vi "DSF.Engine.Plugin.Start.vi"(8 "error in (no error)":errorcluster, 11 "Plugin in":refnum<class "DSF.Engine.Plugin.lvclass">) -> (0 "error out":errorcluster, 3 "Plugin out":refnum<class "DSF.Engine.Plugin.lvclass">)   [LabVIEW 2017, in "DSF.Engine.lvlib" / "DSF.Engine.Plugin.lvclass"]
uses:
  DSF.Engine.Plugin.lvclass
  DSF.Engine.Plugin.lvclass/DSF.Engine.Plugin.ctl
  Timing/DSF.Engine.Timing.lvclass/DSF.Engine.Timing.ctl
  Transceiver/DSF.Engine.Transceiver Thread.lvclass
  Thread Pool/DSF.Engine.Pool.ID.lvclass
  Thread Parameters/Thread Parameters.lvclass
  Timing/DSF.Engine.Timing.lvclass
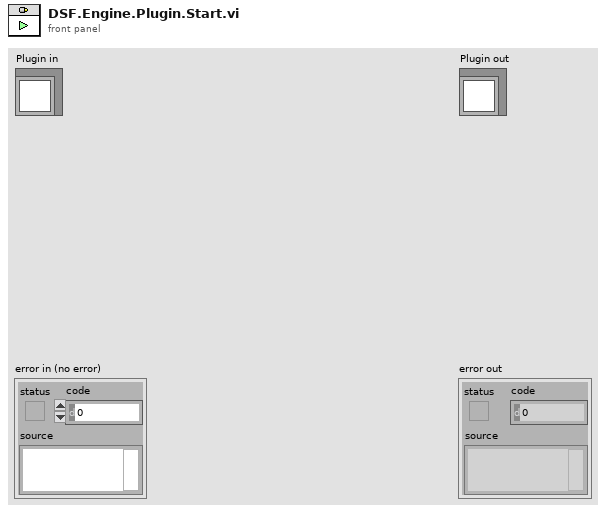
[diagram p1: front panel]
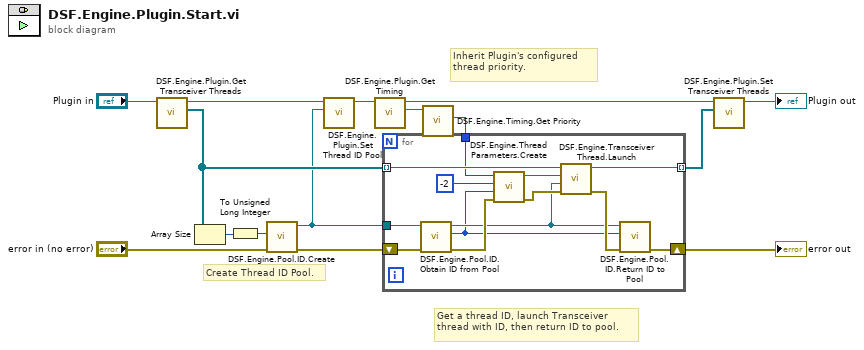
[diagram p0: block diagram]
diagram:
  # "Inherit Plugin's configured thread priority."
  # "Get a thread ID, launch Transceiver thread with ID, then return ID to pool."
  # "Create Thread ID Pool."
  n1 = call "DSF.Engine.Plugin.Get Transceiver Threads.vi"("Plugin in"="Plugin in") -> ("Transceivers"=w11:refnum<class "DSF.Engine.Transceiver Thread.lvclass">[], "Plugin out"=w8:refnum<class "DSF.Engine.Plugin.lvclass">)  [unwired: 9 in]
  n2 = Array Size(array=w11) -> (size(s)=w6:i32)
  n3 = To Unsigned Long Integer(number=w6) -> (unsigned 32bit integer=w5:u32)
  n4 = call "DSF.Engine.Pool.ID.Create.vi"("error in (no error)"="error in (no error)", "number of IDs"=w5) -> ("error out"=w10:errorcluster, "ID Pool out"=w7:refnum<class "DSF.Engine.Pool.ID.lvclass">)  [unwired: 8 in]
  n5 = call "DSF.Engine.Plugin.Set Thread ID Pool.vi"("Thread ID Pool"=w7, "Plugin in"=w8) -> ("Plugin out"=w4:refnum<class "DSF.Engine.Plugin.lvclass">)  [unwired: 9 in]
  n6 = call "DSF.Engine.Plugin.Get Timing.vi"("Plugin in"=w4) -> ("Timing"=w3:refnum<class "DSF.Engine.Timing.lvclass">, "Plugin out"=w1:refnum<class "DSF.Engine.Plugin.lvclass">)  [unwired: 9 in]
  n7 = call "DSF.Engine.Timing.Get Priority.vi"("Timing in"=w3) -> ("Priority"=w2:u64)  [unwired: 9 in, 1 out]
  n8 = for {
    tunnel: [w28] -> w14 mode=indexing
    shift-right: [w20] -> w13
    shift-left: w10 -> [w24]
    tunnel: w11 -> [w27] mode=indexing
    tunnel: w7 -> [w26]
    tunnel: w2 -> [w17]
    n9 = call "DSF.Engine.Pool.ID.Obtain ID from Pool.vi"("error in (no error)"=w24, "ID Pool in"=w26) -> ("error out"=w23:errorcluster, "id"=w16:i32, "ID Pool out"=w19:refnum<class "DSF.Engine.Pool.ID.lvclass">)  [unwired: 6 in, 1 out]
    n10 = call "DSF.Engine.Thread Parameters.Create.vi"("error in (no error)"=w23, "id"=w16, "processor"=-2, "priority"=w17) -> ("error out"=w22:errorcluster, "Thread Parameters"=w18:refnum<class "Thread Parameters.lvclass">)  [unwired: 6 in]
    n11 = call "DSF.Engine.Transceiver Thread.Launch.vi"("error in (no error)"=w22, "Thread ID Pool"=w19, "Thread Parameters"=w18, "Transceiver Thread in"=w27) -> ("error out"=w21:errorcluster, "Transceiver Thread out"=w28:refnum<class "DSF.Engine.Transceiver Thread.lvclass">)  [unwired: 6 in]
    n12 = call "DSF.Engine.Pool.ID.Return ID to Pool.vi"("error in (no error)"=w21, "id"=w16, "ID Pool in"=w19) -> ("error out"=w20:errorcluster)  [unwired: 6 in, 2 out]
  }
  "error out" <- w13
  n13 = call "DSF.Engine.Plugin.Set Transceiver Threads.vi"("Transceivers"=w14, "Plugin in"=w1) -> ("Plugin out"=→"Plugin out":refnum<class "DSF.Engine.Plugin.lvclass">)  [unwired: 9 in]
